vi "String to Bool.vi"(11 "String":string) -> (3 "Bool":bool)   [LabVIEW 2017]
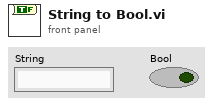
[diagram p1: front panel]
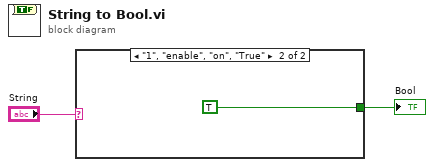
[diagram p0: block diagram]
diagram:
  n1 = case shown="\"1\", \"enable\", \"on\", \"True\"" "String" {
    tunnel: [_ TRUE ("Front Panel Window:Show Menu Bar")] -> w2
    frame "", "0", "Disable", "False", "off", Default {
    }
    frame "1", "enable", "on", "True" {
    }
  }
  "Bool" <- w2
